vi "Get Datetime Format.vi"(8 "error in":errorcluster, 11 "Formatter in":refnum<class "Formatter.lvclass">) -> (0 "error out":errorcluster, 2 "Datetime Format":string="%Y-%m-%d %H:%M:%S", 3 "Formatter out":refnum<class "Formatter.lvclass">)   [LabVIEW 2024, in "hse-logger.lvlib" / "Formatter.lvclass"]
doc: "Returns the date/time format used to format a timestamp using the Format Date/Time String function.\n\n____\nHAMPEL SOFTWARE ENGINEERING v2.2.2 (2025-01-16 15:41)"
uses:
  <vilib>/Hampel Software Engineering/HSE Logger/Formatter/Formatter.lvclass
  <vilib>/Hampel Software Engineering/HSE Logger/Formatter/Formatter.lvclass/Formatter.ctl
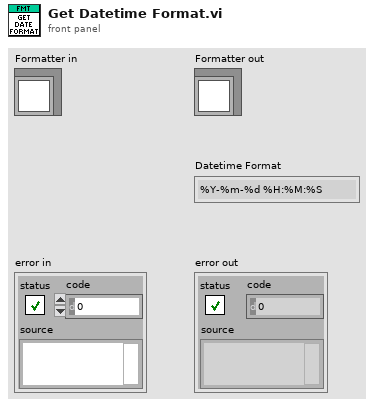
[diagram p1: front panel]
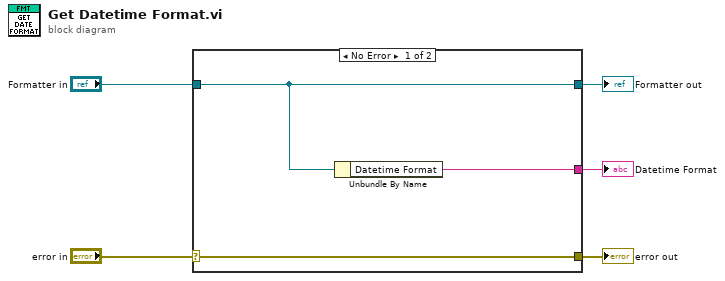
[diagram p0: block diagram]
diagram:
  n1 = case shown="No Error" "error in" {
    selector: "error in" -> [w8 w10]
    tunnel: [w8 w10] -> w4
    tunnel: [w7 w9] -> w2
    tunnel: "Formatter in" -> [w7 w9]
    tunnel: [w6 _] -> w1
    frame No Error {
      n2 = Unbundle By Name(w7) -> ("Datetime Format"=w6:string)
    }
    frame Error {
    }
  }
  "error out" <- w4
  "Formatter out" <- w2
  "Datetime Format" <- w1
